vi "Instrument Manager Loop.vi"(8 "System Control":refnum<queue>, 11 "Instrument Manager":refnum<queue>) -> (0 "error out":errorcluster)   [LabVIEW 2020, in "plugin_flodx_pressure.lvlib" / "plugin.lvlib" / "Instrument Manager.lvlib"]
uses:
  Instrument Manager.lvlib
  <userlib>/RxnRover/PluginCore/src/support/Message Queue/Message Cluster.ctl
  Instrument Loop State.ctl
  connection_info/Connection Info.ctl
  Instrument State.ctl
  Instrument Config.ctl
  <vilib>/Utility/error.llb/Error Cluster From Error Code.vi
  <vilib>/ErrorRing/Error Ring.xnode
  <userlib>/RxnRover/PluginCore/src/support/Message Queue/Message Queue.lvlib
  <userlib>/_OpenG.lib/lvdata/lvdata.llb/openg_variant.lvlib
  mock_driver/mock_driver.lvlib
  <instrlib>/RxnRover/FloDx Pressure Driver/driver_flodx_pressure.lvlib
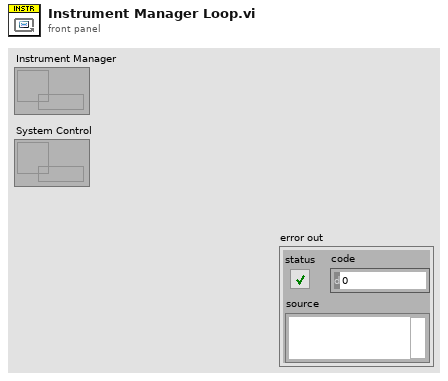
[diagram p1: front panel]
types:
  T1 = typedef "plugin_flodx_pressure.lvlib/plugin.lvlib/Instrument Manager.lvlib/Instrument Loop State.ctl" = cluster{"Connection Info":T2, "Running":bool, "Running Since":timestamp, "Instrument State":T3}
  T2 = typedef "plugin_flodx_pressure.lvlib/plugin.lvlib/Instrument Manager.lvlib/Connection Info.ctl" = cluster{"VISA Resource":refnum<visa-resource-name>, "Address":u8}
  T3 = typedef "plugin_flodx_pressure.lvlib/plugin.lvlib/Instrument Manager.lvlib/Instrument State.ctl" = cluster{"Abs. Pressure":sgl, "Amb. Pressure":sgl, "Device":string, "Firmware Version":string, "Error Status":bool, "Error Code":i32, "Error Source":string, "Gauge Pressure":sgl, "Temperature":sgl, "Units (0-kPa,1-PSI,2-BAR)":dbl}
  T4 = typedef "plugin_flodx_pressure.lvlib/plugin.lvlib/Instrument Manager.lvlib/Instrument Config.ctl" = cluster{"Device":string, "Firmware Version":string}
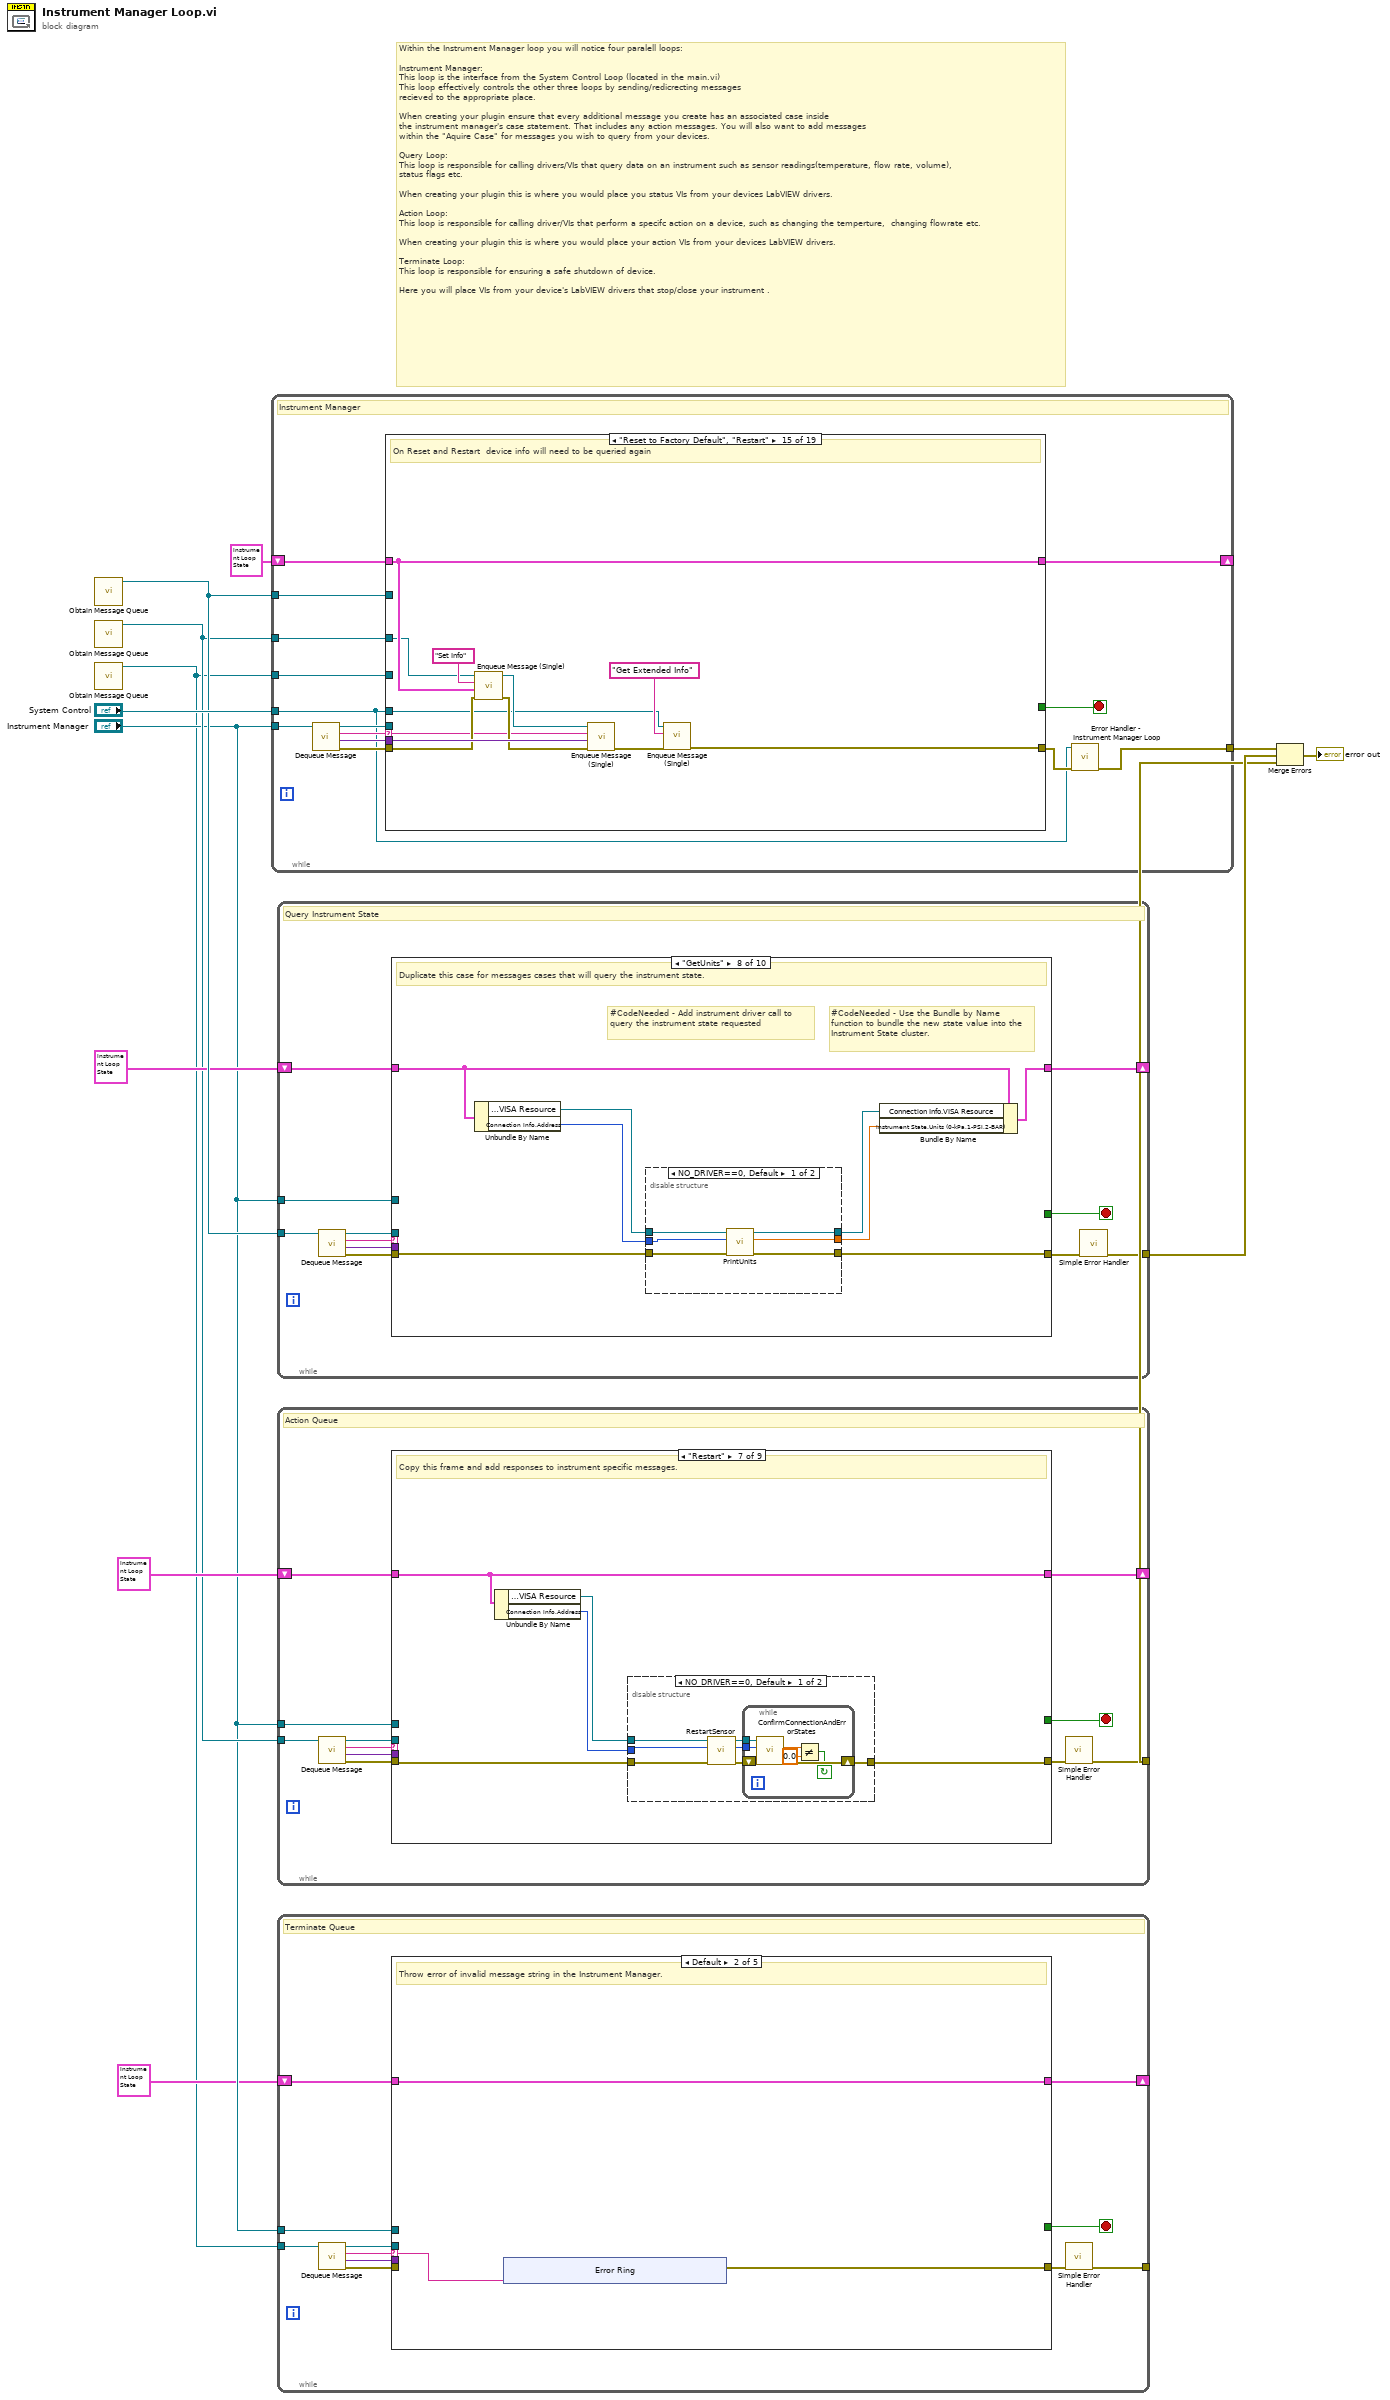
[diagram p0: block diagram]
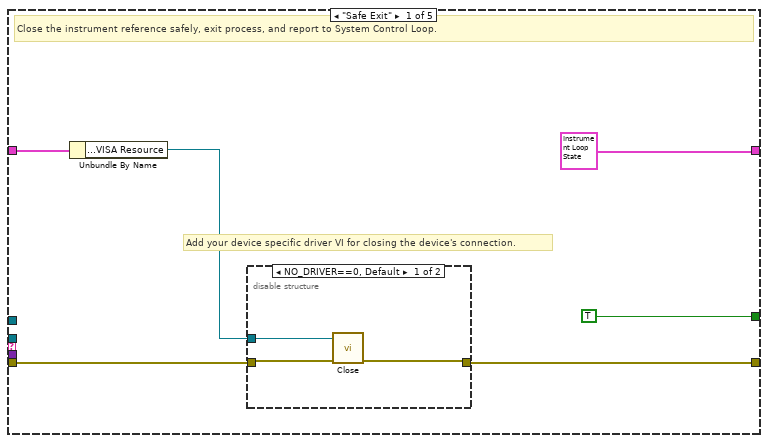
[diagram p2: hidden frame]
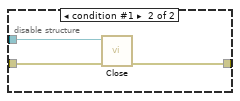
[diagram p3: hidden frame]
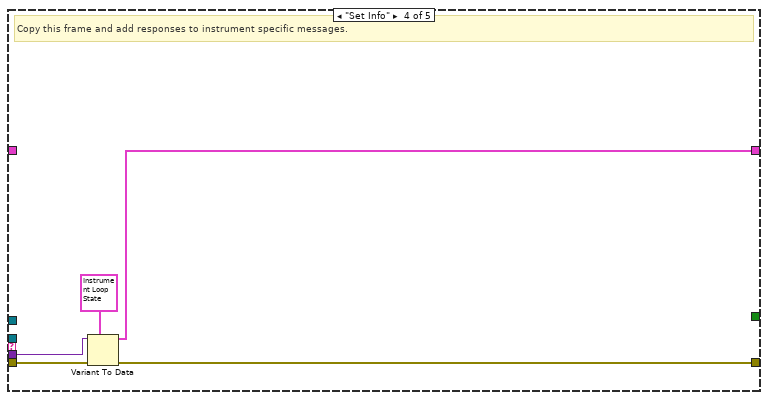
[diagram p5: hidden frame]
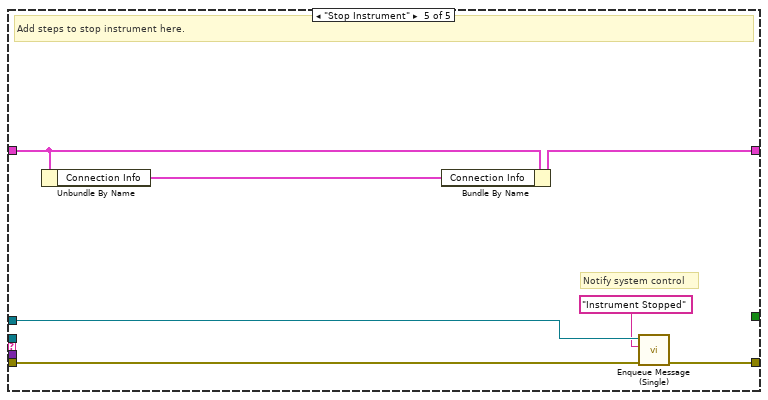
[diagram p6: hidden frame]
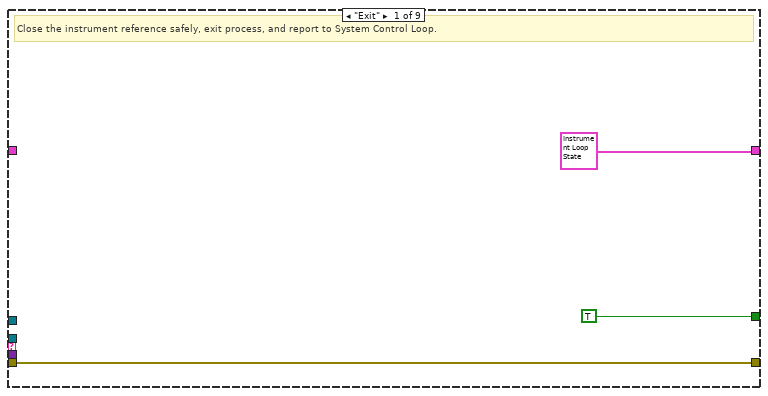
[diagram p7: hidden frame]
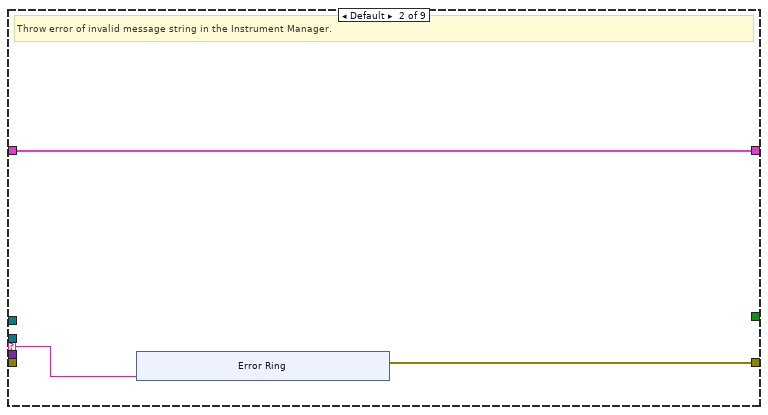
[diagram p8: hidden frame]
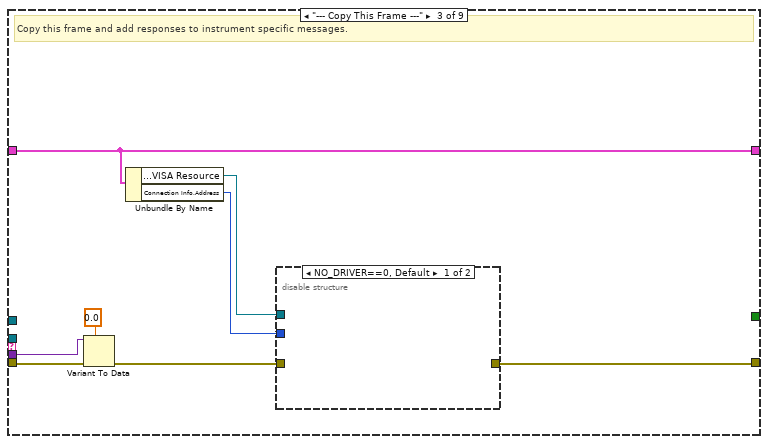
[diagram p9: hidden frame]
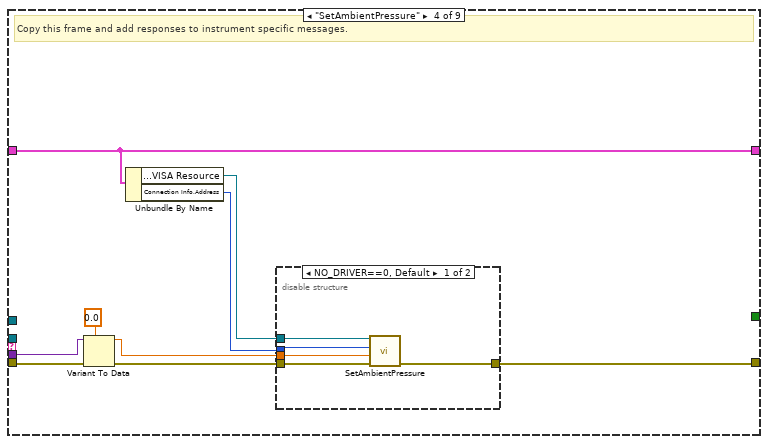
[diagram p11: hidden frame]
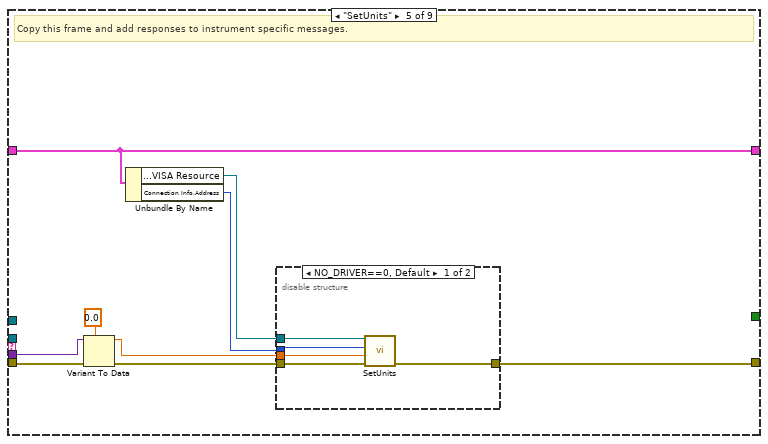
[diagram p13: hidden frame]
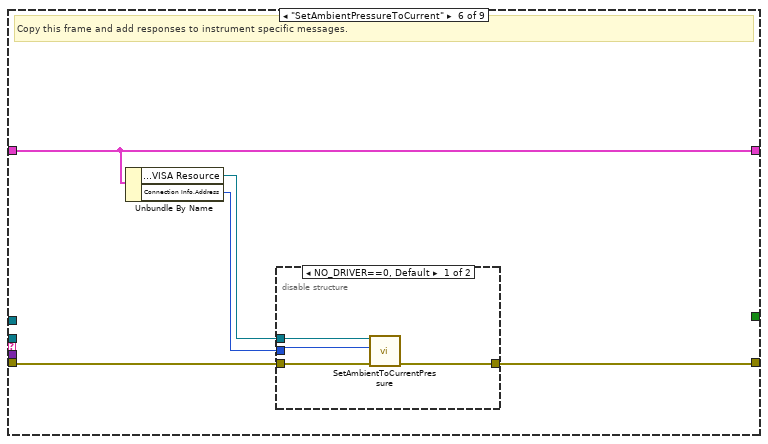
[diagram p15: hidden frame]
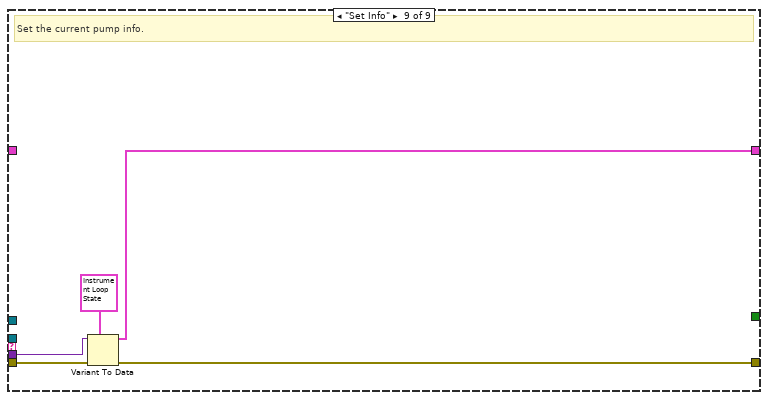
[diagram p19: hidden frame]
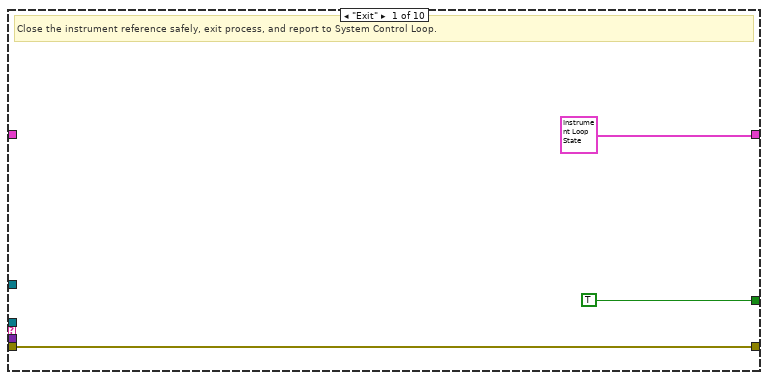
[diagram p20: hidden frame]
diagram:
  # "Within the Instrument Manager loop you will notice four paralell loops:\n\nInstrument Manager:\nThis loop is the interface from the System Control Loop (located in the main.vi)\nThis loop effectively controls the other three loops by sending/redicrecting messages\nrecieved to the appropriate place. \n\nWhen creating your plugin ensure that every additional message you create has an associated case inside \nthe instrument manager's case statement. That includes any action messages. You will also want to add messages\nwithin the \"Aquire Case\" for messages you wish to query from your devices.\n\nQuery Loop:\nThis loop is responsible for calling drivers/VIs that query data on an instrument such as sensor readings(temperature, flow rate, volume),\nstatus flags etc.\n\nWhen creating your plugin this is where you would place you status VIs from your devices LabVIEW drivers.\n\nAction Loop: \nThis loop is responsible for calling driver/VIs that perform a specifc action on a device, such as changing the temperture,  changing flowrate etc.\n\nWhen creating your plugin this is where you would place your action VIs from your devices LabVIEW drivers.\n\nTerminate Loop:\nThis loop is responsible for ensuring a safe shutdown of device. \n\nHere you will place VIs from your device's LabVIEW drivers that stop/close your instrument ."
  n1 = call <userlib>:"Obtain Message Queue.vi"() -> ("Message Queue"=w10:refnum<queue>)  [unwired: 10 in, 1 out]
  n2 = call <userlib>:"Obtain Message Queue.vi"() -> ("Message Queue"=w5:refnum<queue>)  [unwired: 10 in, 1 out]
  n3 = call <userlib>:"Obtain Message Queue.vi"() -> ("Message Queue"=w1:refnum<queue>)  [unwired: 10 in, 1 out]
  n4 = while {
    tunnel: "Instrument Manager" -> [w27]
    tunnel: "System Control" -> [w18]
    tunnel: [w21] -> w13
    shift-right: [w14] -> _
    shift-left: T1 {"Connection Info"={"VISA Resource"="", "Address"=1}, "Running"=FALSE, "Running Since"=timestamp(0 s since 1904-01-01), "Instrument State"={"Abs. Pressure"=0.0, "Amb. Pressure"=0.0, "Device"="", "Firmware Version"="", "Error Status"=FALSE, "Error Code"=0, "Error Source"="", "Gauge Pressure"=0.0, "Temperature"=0.0, "Units (0-kPa,1-PSI,2-BAR)"=0.0}} ("Default Instrument State") -> [w20]
    tunnel: w10 -> [w17]
    tunnel: w5 -> [w16]
    tunnel: w1 -> [w15]
    stop <- w19 stop-if-true
    # "Instrument Manager"
    n5 = call <userlib>:"Dequeue Message.vi"("Message Queue"=w27) -> ("error out"=w23:errorcluster, "Message Data"=w24:variant, "Message"=w26:string, "dup Message Queue"=w25:refnum<queue>)  [unwired: 7 in]
    n6 = case shown="\"Reset to Factory Default\", \"Restart\"" w26 {
      selector: w26 -> [_ w37 _ _ _ _ _ w83 _ _ w128 w132 w145 w154 w167 _ _ _ _]
      tunnel: w25 -> [w30 _ _ w54 _ _ _ _ _ w94 _ _ _ _ _ _ _ _ w206]
      tunnel: w18 -> [_ w38 _ _ w64 w74 w80 _ _ w96 w124 _ _ _ w162 _ _ _ _]
      tunnel: w24 -> [_ _ _ w61 _ _ _ _ _ w102 w127 w139 w151 w160 w173 _ _ _ w207]
      tunnel: w23 -> [w31 w39 w46 w59 w66 w71 w77 _ w92 w101 w126 w136 w148 w157 w170 w175 w176 w192 w212]
      tunnel: [w29 w33 w47 w56 w65 w75 w81 w82 w92 w105 w129 w140 w152 w161 w164 w175 w182 w202 w203] -> w22
      tunnel: w20 -> [_ w36 _ w60 w67 w69 w78 w84 w93 w104 w125 w137 w149 w158 w171 w174 w181 w199 w211]
      tunnel: [w32 w36 T1 {"Connection Info"={"VISA Resource"="", "Address"=1}, "Running"=FALSE, "Running Since"=timestamp(0 s since 1904-01-01), "Instrument State"={"Abs. Pressure"=0.0, "Amb. Pressure"=0.0, "Device"="", "Firmware Version"="", "Error Status"=FALSE, "Error Code"=0, "Error Source"="", "Gauge Pressure"=0.0, "Temperature"=0.0, "Units (0-kPa,1-PSI,2-BAR)"=0.0}} w60 w67 w69 w78 w84 w93 w103 w125 w131 w144 w158 w171 w174 w181 w199 w205] -> w14
      tunnel: [_ _ TRUE _ _ _ _ _ _ _ _ _ _ _ _ _ _ _ _] -> w19
      tunnel: w17 -> [_ _ w41 _ _ _ _ _ _ _ _ _ _ _ _ _ w180 w194 _]
      tunnel: w16 -> [_ _ w42 _ _ _ _ _ _ _ _ _ w141 w153 w166 _ _ _ _]
      tunnel: w15 -> [_ _ w43 _ _ _ _ _ _ _ _ w134 _ _ _ _ _ _ _]
      frame "Initialize" {
        (unwired) string[] ["Send Instrument Config", "Send Entry Names"]
        w32 = T1 {"Connection Info"={"VISA Resource"="", "Address"=1}, "Running"=FALSE, "Running Since"=timestamp(0 s since 1904-01-01), "Instrument State"={"Abs. Pressure"=0.0, "Amb. Pressure"=0.0, "Device"="", "Firmware Version"="", "Error Status"=FALSE, "Error Code"=0, "Error Source"="", "Gauge Pressure"=0.0, "Temperature"=0.0, "Units (0-kPa,1-PSI,2-BAR)"=0.0}}  # Default Instrument State
        # "Initialize the loop data."
        n7 = call <userlib>:"Enqueue Message (Array).vi"("error in (no error)"=w31, "Message Array"=string[] ["Send Instrument Config", "Send Acquisition Messages", "Send Entry Names"], "Message Queue"=w30) -> ("error out"=w29:errorcluster)  [unwired: 7 in, 1 out]
      }
      frame "Report" {
        # "Reports the instrument state to the system control loop to populate the rest of the plugin"
        # "Unblock querying"
        # "Report the instrument state."
        n8 = call <userlib>:"Enqueue Message (Single).vi"("error in (no error)"=w39, "Message Data"=w36, "Message"=w37, "Message Queue"=w38) -> ("error out"=w34:errorcluster)  [unwired: 6 in, 1 out]
        n9 = call "QueryInProgress.vi"("error in (no error)"=w34, "Action"=enum16{"Get", "Set False", "Set True"}."Set False") -> ("error out"=w33:errorcluster)  [unwired: 8 in, 1 out]
      }
      frame "Exit" {
        # "Close the instrument reference safely, exit process, and report to System Control Loop."
        n10 = Build Array(w41, w42) -> (w40:refnum<queue>[])
        n11 = call <userlib>:"Enqueue Message (Single).vi"("error in (no error)"=w46, "Message"="Safe Exit", "Message Queue"=w43) -> ("error out"=w45:errorcluster)  [unwired: 7 in, 1 out]
        n12 = for {
          tunnel: w40 -> [w52] mode=indexing
          tunnel: w45 -> [w50]
          tunnel: [w53] -> w47
          n13 = call <userlib>:"Enqueue Message (Single).vi"("error in (no error)"=w50, "Message"="Exit", "Message Queue"=w52) -> ("error out"=w53:errorcluster)  [unwired: 7 in, 1 out]
        }
      }
      frame "New Instrument Config" {
        # "No settings right now"
        # "If the new config is accepted, notify everything of the new values"
        # "Update the configs based on the user settings."
        n14 = Variant To Data(error in=w59, type=T4 {"Device"="", "Firmware Version"=""} ("Instrument Configuration"), Variant=w61) -> (error out=w55:errorcluster)  [unwired: 1 out]
        n15 = call <userlib>:"Enqueue Message (Single).vi"("error in (no error)"=w55, "Message"="Send Instrument Config", "Message Queue"=w54) -> ("error out"=w56:errorcluster)  [unwired: 7 in, 1 out]
      }
      frame "Send Instrument Config" {
        # "Send out the current values for the public loop configs."
        n16 = call <userlib>:"Enqueue Message (Single).vi"("error in (no error)"=w66, "Message Data"=T4 {"Device"="", "Firmware Version"=""} ("Instrument Configuration"), "Message"="Instrument Config", "Message Queue"=w64) -> ("error out"=w65:errorcluster)  [unwired: 6 in, 1 out]
      }
      frame "Send Entry Names" {
        # "#note: This is auto-populated based on the Instrument State TypeDef entry labels."
        # "Send the display names of entry values that will be reported by this instrument in each \"Report\" call."
        n17 = Unbundle By Name(w69) -> ("Instrument State"=w68:T3)
        n18 = call <userlib>:"Get Cluster Element Names__ogtk.vi"("error in (no error)"=w71, "Cluster"=w68) -> ("error out"=w70:errorcluster, "Element Names"=w72:string[])  [unwired: 8 in]
        n19 = call <userlib>:"Enqueue Message (Single).vi"("error in (no error)"=w70, "Message Data"=w72, "Message"="Set Entry Names", "Message Queue"=w74) -> ("error out"=w75:errorcluster)  [unwired: 6 in, 1 out]
      }
      frame "Send Acquisition Messages" {
        # "Send the messages that should be used to acquire the relevant instrument state and how to report it."
        n20 = call <userlib>:"Enqueue Message (Single).vi"("error in (no error)"=w77, "Message Data"=string[] ["Acquire"], "Message"="Set Acquisition Messages", "Message Queue"=w80) -> ("error out"=w81:errorcluster)  [unwired: 6 in, 1 out]
      }
      frame Default {
        # "Throw error of invalid message string in the Instrument Manager."
        n21 = xnode "Error Ring"("parameter 0"=w83) -> ("error out"=w82:errorcluster)
      }
      frame "--- Copy This Frame ---" {
        # "Copy this frame and add responses to instrument specific messages."
      }
      frame "Set Connection Info" {
        # "Validate and initialize the connection info"
        n22 = Variant To Data(error in=w101, type=T2 {"VISA Resource"="", "Address"=1} ("Connection Info"), Variant=w102) -> (data=w99:T2, error out=w100:errorcluster)
        n23 = call "Attempt Connection.vi"("error in (no error)"=w100, "Connection Info"=w99) -> ("error out"=w97:errorcluster, "Connection Info (duplicate)"=w98:T2)  [unwired: 8 in]
        n24 = case shown="No Error" w97 {
          selector: w97 -> [w107 w119]
          tunnel: w98 -> [w106 _]
          tunnel: [w108 w122] -> w105
          tunnel: w104 -> [w115 w123]
          tunnel: [w117 w123] -> w103
          tunnel: w96 -> [w116 w121]
          tunnel: w94 -> [w112 _]
          frame No Error {
            # "Notify System Control of valid connection info"
            # "Initialize valid resource."
            n25 = call <userlib>:"Enqueue Message (Single).vi"("error in (no error)"=w107, "Message Data"=w106, "Message"="Valid Connection Info", "Message Queue"=w116) -> ("error out"=w114:errorcluster)  [unwired: 6 in, 1 out]
            n26 = Bundle By Name(cluster=w115, "Connection Info"=w106) -> (w117:T1)
            n27 = call <userlib>:"Enqueue Message (Single).vi"("error in (no error)"=w114, "Message"="Send Acquisition Messages", "Message Queue"=w112) -> ("error out"=w109:errorcluster, "dup Message Queue"=w111:refnum<queue>)  [unwired: 7 in]
            n28 = call <userlib>:"Enqueue Message (Single).vi"("error in (no error)"=w109, "Message"="Get Extended Info", "Message Queue"=w111) -> ("error out"=w108:errorcluster)  [unwired: 7 in, 1 out]
          }
          frame Error {
            # "Report invalid resource."
            n29 = call <userlib>:"Enqueue Message (Single).vi"("Message Data"=w119, "Message"="Invalid Connection Info", "Message Queue"=w121) -> ("error out"=w122:errorcluster)  [unwired: 7 in, 1 out]
          }
        }
      }
      frame "Instrument Started", "Instrument Stopped" {
        # "Forward start/stop messages to the rest of the program."
        n30 = call <userlib>:"Enqueue Message (Single).vi"("error in (no error)"=w126, "Message Data"=w127, "Message"=w128, "Message Queue"=w124) -> ("error out"=w129:errorcluster)  [unwired: 6 in, 1 out]
      }
      frame "Stop Instrument" {
        # "Stop the instrument action."
        n31 = call <userlib>:"Enqueue Message (Single).vi"("error in (no error)"=w136, "Message Data"=w137, "Message"="Set Info", "Message Queue"=w134) -> ("error out"=w135:errorcluster, "dup Message Queue"=w133:refnum<queue>)  [unwired: 6 in]
        n32 = call <userlib>:"Enqueue Message (Single).vi"("error in (no error)"=w135, "Message Data"=w139, "Message"=w132, "Message Queue"=w133) -> ("error out"=w140:errorcluster)  [unwired: 6 in, 1 out]
        n33 = Bundle By Name(cluster=w137, "Running"=FALSE) -> (w131:T1)
      }
      frame "Start Instrument" {
        # "Start the instrument action."
        n34 = call <userlib>:"Enqueue Message (Single).vi"("error in (no error)"=w148, "Message Data"=w149, "Message"="Set Info", "Message Queue"=w141) -> ("error out"=w147:errorcluster, "dup Message Queue"=w146:refnum<queue>)  [unwired: 6 in]
        n35 = call <userlib>:"Enqueue Message (Single).vi"("error in (no error)"=w147, "Message Data"=w151, "Message"=w145, "Message Queue"=w146) -> ("error out"=w152:errorcluster)  [unwired: 6 in, 1 out]
        n36 = Get Date/Time In Seconds() -> (seconds since 1Jan1904=w142:timestamp)
        n37 = Bundle By Name(cluster=w149, "Running"=TRUE, "Running Since"=w142) -> (w144:T1)
      }
      frame "SetAmbientPressure", "SetAmbientPressureToCurrent", "SetUnits" {
        # "Actions to be forwarded to the Action loop"
        n38 = call <userlib>:"Enqueue Message (Single).vi"("error in (no error)"=w157, "Message Data"=w158, "Message"="Set Info", "Message Queue"=w153) -> ("error out"=w156:errorcluster, "dup Message Queue"=w155:refnum<queue>)  [unwired: 6 in]
        n39 = call <userlib>:"Enqueue Message (Single).vi"("error in (no error)"=w156, "Message Data"=w160, "Message"=w154, "Message Queue"=w155) -> ("error out"=w161:errorcluster)  [unwired: 6 in, 1 out]
      }
      frame "Reset to Factory Default", "Restart" {
        # "On Reset and Restart  device info will need to be queried again"
        n40 = call <userlib>:"Enqueue Message (Single).vi"("error in (no error)"=w170, "Message Data"=w171, "Message"="Set Info", "Message Queue"=w166) -> ("error out"=w169:errorcluster, "dup Message Queue"=w168:refnum<queue>)  [unwired: 6 in]
        n41 = call <userlib>:"Enqueue Message (Single).vi"("error in (no error)"=w169, "Message Data"=w173, "Message"=w167, "Message Queue"=w168) -> ("error out"=w165:errorcluster)  [unwired: 6 in, 1 out]
        n42 = call <userlib>:"Enqueue Message (Single).vi"("error in (no error)"=w165, "Message"="Get Extended Info", "Message Queue"=w162) -> ("error out"=w164:errorcluster)  [unwired: 7 in, 1 out]
      }
      frame "--- Copy for Get State Messages ---" {
        # "#CodeNeeded - Use the Bundle by Name function to bundle the new state value into the Instrument State cluster."
        # "#CodeNeeded - Add instrument driver call to query the instrument state requested"
        # "Duplicate this case for messages cases that will query the instrument state."
      }
      frame "Acquire" {
        # "Only query if there isn't another query in progress"
        # "Query the run state of the instrument."
        n43 = call "QueryInProgress.vi"("error in (no error)"=w176, "Action"=enum16{"Get", "Set False", "Set True"}."Get") -> ("error out"=w177:errorcluster, "Value"=w178:bool)  [unwired: 8 in]
        n44 = case shown="False" w178 {
          tunnel: w177 -> [w183 w191]
          tunnel: [w183 w190] -> w182
          tunnel: w181 -> [_ w187]
          tunnel: w180 -> [_ w185]
          frame True {
            # "There is another process inside Query Instrument\nstate, wait until it is finished"
          }
          frame False {
            # "replace this and add more\nif needed"
            n45 = call <userlib>:"Enqueue Message (Single).vi"("error in (no error)"=w191, "Message Data"=w187, "Message"="Set Info", "Message Queue"=w185) -> ("error out"=w188:errorcluster, "dup Message Queue"=w184:refnum<queue>)  [unwired: 6 in]
            n46 = call <userlib>:"Enqueue Message (Array).vi"("error in (no error)"=w188, "Message Array"=string[] ["GetGaugePressure", "GetAbsolutePressure", "GetTemperature", "Send Instr State"], "Message Queue"=w184) -> ("error out"=w190:errorcluster)  [unwired: 7 in, 1 out]
          }
        }
      }
      frame "Get Extended Info" {
        # "Add query messages to get\nimportant information but \nnot necessarilly required \nqueried constantly, such as\ndevice firmware information,\nname, etc."
        # "Block Aquire from querying"
        # "This is high priority, and is non-blocked from querying instrument state"
        # "This is information that is important but not necessarily required to be queried every time aquire message is sent"
        n47 = Flush Queue(queue=w194) -> (queue out=w193:refnum<queue>)  [unwired: 1 in, 2 out]
        n48 = call "QueryInProgress.vi"("error in (no error)"=w192, "Action"=enum16{"Get", "Set False", "Set True"}."Set True") -> ("error out"=w195:errorcluster)  [unwired: 8 in, 1 out]
        n49 = call <userlib>:"Enqueue Message (Single).vi"("error in (no error)"=w195, "Message Data"=w199, "Message"="Set Info", "Message Queue"=w193) -> ("error out"=w200:errorcluster, "dup Message Queue"=w197:refnum<queue>)  [unwired: 6 in]
        n50 = call <userlib>:"Enqueue Message (Array).vi"("error in (no error)"=w200, "Message Array"=string[] ["GetUnits", "GetAmbientPressure", "Send Instr State"], "Message Queue"=w197) -> ("error out"=w202:errorcluster)  [unwired: 7 in, 1 out]
      }
      frame "Set Instr State" {
        # "Set the new instrument state queried from the instrument."
        n51 = Variant To Data(error in=w212, type=T3 {"Abs. Pressure"=0.0, "Amb. Pressure"=0.0, "Device"="", "Firmware Version"="", "Error Status"=FALSE, "Error Code"=0, "Error Source"="", "Gauge Pressure"=0.0, "Temperature"=0.0, "Units (0-kPa,1-PSI,2-BAR)"=0.0} ("Instrument State"), Variant=w207) -> (data=w204:T3, error out=w209:errorcluster)
        n52 = Bundle By Name(cluster=w211, "Instrument State"=w204) -> (w205:T1)
        n53 = call <userlib>:"Enqueue Message (Single).vi"("error in (no error)"=w209, "Message"="Report", "Message Queue"=w206) -> ("error out"=w203:errorcluster)  [unwired: 7 in, 1 out]
      }
    }
    n54 = call "Error Handler - Instrument Manager Loop.vi"("error in (no error)"=w22, "Message Queue"=w18) -> ("dup error in"=w21:errorcluster)  [unwired: 8 in, 1 out]
  }
  n55 = while {
    tunnel: w10 -> [w223]
    shift-right: [w217] -> _
    shift-left: T1 {"Connection Info"={"VISA Resource"="", "Address"=1}, "Running"=FALSE, "Running Since"=timestamp(0 s since 1904-01-01), "Instrument State"={"Abs. Pressure"=0.0, "Amb. Pressure"=0.0, "Device"="", "Firmware Version"="", "Error Status"=FALSE, "Error Code"=0, "Error Source"="", "Gauge Pressure"=0.0, "Temperature"=0.0, "Units (0-kPa,1-PSI,2-BAR)"=0.0}} ("Default Instrument State") -> [w218]
    tunnel: "Instrument Manager" -> [w215]
    tunnel: [w213] -> w7
    stop <- w216 stop-if-true
    # "Query Instrument State"
    n56 = call <userlib>:"Dequeue Message.vi"("Message Queue"=w223) -> ("error out"=w219:errorcluster, "Message Data"=w220:variant, "Message"=w222:string, "dup Message Queue"=w221:refnum<queue>)  [unwired: 7 in]
    n57 = case shown="\"GetUnits\"" w222 {
      selector: w222 -> [_ w228 _ _ _ _ _ _ _ _]
      tunnel: w221 -> [_ _ _ _ _ _ _ _ _ _]
      tunnel: w220 -> [_ _ _ _ _ _ _ _ w331 _]
      tunnel: w219 -> [w224 _ w241 w250 w267 w284 w301 w318 w333 w339]
      tunnel: [w224 w227 w242 w251 w268 w285 w302 w319 w332 w334] -> w214
      tunnel: w218 -> [_ w229 w239 w248 w265 w282 w299 w316 _ w337]
      tunnel: [T1 {"Connection Info"={"VISA Resource"="", "Address"=1}, "Running"=FALSE, "Running Since"=timestamp(0 s since 1904-01-01), "Instrument State"={"Abs. Pressure"=0.0, "Amb. Pressure"=0.0, "Device"="", "Firmware Version"="", "Error Status"=FALSE, "Error Code"=0, "Error Source"="", "Gauge Pressure"=0.0, "Temperature"=0.0, "Units (0-kPa,1-PSI,2-BAR)"=0.0}} w229 w240 w249 w266 w283 w300 w317 w329 w337] -> w217
      tunnel: [TRUE _ _ _ _ _ _ _ _ _] -> w216
      tunnel: w215 -> [_ _ _ _ _ _ _ _ _ w338]
      frame "Exit" {
        # "Close the instrument reference safely, exit process, and report to System Control Loop."
      }
      frame Default {
        # "Throw error of invalid message string in the Instrument Manager."
        n58 = xnode "Error Ring"("parameter 0"=w228) -> ("error out"=w227:errorcluster)
      }
      frame "--- Copy for Get State Messages ---" {
        # "#CodeNeeded - Use the Bundle by Name function to bundle the new state value into the Instrument State cluster."
        # "#CodeNeeded - Add instrument driver call to query the instrument state requested"
        # "Duplicate this case for messages cases that will query the instrument state."
        n59 = Unbundle By Name(w239) -> ("Connection Info.VISA Resource"=w238:refnum<visa-resource-name>)  [unwired: 2 out]
        n60 = disable-structure shown="NO_DRIVER==0, Default" {
          disable-tunnel: w241 -> [_ w243]
          disable-tunnel: [_ w243] -> w242
          disable-tunnel: w238 -> [_ _]
          frame condition #0 (active) {
          }
          frame condition #1 {
          }
        }
        n61 = Bundle By Name(cluster=w239, "Instrument State"=T3 {"Abs. Pressure"=0.0, "Amb. Pressure"=0.0, "Device"="", "Firmware Version"="", "Error Status"=FALSE, "Error Code"=0, "Error Source"="", "Gauge Pressure"=0.0, "Temperature"=0.0, "Units (0-kPa,1-PSI,2-BAR)"=0.0}) -> (w240:T1)
      }
      frame "GetAmbientPressure" {
        # "#CodeNeeded - Use the Bundle by Name function to bundle the new state value into the Instrument State cluster."
        # "#CodeNeeded - Add instrument driver call to query the instrument state requested"
        # "Duplicate this case for messages cases that will query the instrument state."
        n62 = Unbundle By Name(w248) -> ("Connection Info.VISA Resource"=w247:refnum<visa-resource-name>, "Connection Info.Address"=w246:u8)
        n63 = disable-structure shown="NO_DRIVER==0, Default" {
          disable-tunnel: w250 -> [w256 w260]
          disable-tunnel: [w257 w260] -> w251
          disable-tunnel: w247 -> [w255 w259]
          disable-tunnel: w246 -> [w254 _]
          disable-tunnel: [w253 21.0 ("Ambient Pressure")] -> w245
          disable-tunnel: [w252 w259] -> w244
          frame condition #0 (active) {
            n64 = call <instrlib>:"PrintAmbientPressure.vi"("error in (no error)"=w256, "Address"=w254, "VISA resource name"=w255) -> ("error out"=w257:errorcluster, "Ambient Pressure"=w253:dbl, "VISA resource name out"=w252:refnum<visa-resource-name>)  [unwired: 5 in, 1 out]
          }
          frame condition #1 {
          }
        }
        n65 = Bundle By Name(cluster=w248, "Connection Info.VISA Resource"=w244, "Instrument State.Amb. Pressure"=w245) -> (w249:T1)
      }
      frame "GetAbsolutePressure" {
        # "#CodeNeeded - Use the Bundle by Name function to bundle the new state value into the Instrument State cluster."
        # "#CodeNeeded - Add instrument driver call to query the instrument state requested"
        # "Duplicate this case for messages cases that will query the instrument state."
        n66 = Unbundle By Name(w265) -> ("Connection Info.VISA Resource"=w264:refnum<visa-resource-name>, "Connection Info.Address"=w263:u8)
        n67 = disable-structure shown="NO_DRIVER==0, Default" {
          disable-tunnel: w267 -> [w273 w277]
          disable-tunnel: [w274 w277] -> w268
          disable-tunnel: w264 -> [w272 w276]
          disable-tunnel: w263 -> [w271 _]
          disable-tunnel: [w270 21.0 ("Ambient Pressure")] -> w262
          disable-tunnel: [w269 w276] -> w261
          frame condition #0 (active) {
            n68 = call <instrlib>:"PrintAbsolutePressure.vi"("error in (no error)"=w273, "Address"=w271, "VISA resource name"=w272) -> ("error out"=w274:errorcluster, "Abs. Pressure"=w270:dbl, "VISA resource name out"=w269:refnum<visa-resource-name>)  [unwired: 5 in, 1 out]
          }
          frame condition #1 {
          }
        }
        n69 = Bundle By Name(cluster=w265, "Connection Info.VISA Resource"=w261, "Instrument State.Abs. Pressure"=w262) -> (w266:T1)
      }
      frame "GetGaugePressure" {
        # "#CodeNeeded - Use the Bundle by Name function to bundle the new state value into the Instrument State cluster."
        # "#CodeNeeded - Add instrument driver call to query the instrument state requested"
        # "Duplicate this case for messages cases that will query the instrument state."
        n70 = Unbundle By Name(w282) -> ("Connection Info.VISA Resource"=w281:refnum<visa-resource-name>, "Connection Info.Address"=w280:u8)
        n71 = disable-structure shown="NO_DRIVER==0, Default" {
          disable-tunnel: w284 -> [w290 w294]
          disable-tunnel: [w291 w294] -> w285
          disable-tunnel: w281 -> [w289 w293]
          disable-tunnel: w280 -> [w288 _]
          disable-tunnel: [w287 21.0 ("Ambient Pressure")] -> w279
          disable-tunnel: [w286 w293] -> w278
          frame condition #0 (active) {
            n72 = call <instrlib>:"PrintGaugePresssure.vi"("error in (no error)"=w290, "Address"=w288, "VISA resource name"=w289) -> ("error out"=w291:errorcluster, "Print Gauge Pressure"=w287:dbl, "VISA resource name out"=w286:refnum<visa-resource-name>)  [unwired: 5 in, 1 out]
          }
          frame condition #1 {
          }
        }
        n73 = Bundle By Name(cluster=w282, "Connection Info.VISA Resource"=w278, "Instrument State.Gauge Pressure"=w279) -> (w283:T1)
      }
      frame "GetTemperature" {
        # "#CodeNeeded - Use the Bundle by Name function to bundle the new state value into the Instrument State cluster."
        # "#CodeNeeded - Add instrument driver call to query the instrument state requested"
        # "Duplicate this case for messages cases that will query the instrument state."
        n74 = Unbundle By Name(w299) -> ("Connection Info.VISA Resource"=w298:refnum<visa-resource-name>, "Connection Info.Address"=w297:u8)
        n75 = disable-structure shown="NO_DRIVER==0, Default" {
          disable-tunnel: w301 -> [w307 w311]
          disable-tunnel: [w308 w311] -> w302
          disable-tunnel: w298 -> [w306 w310]
          disable-tunnel: w297 -> [w305 _]
          disable-tunnel: [w304 21.0 ("Ambient Pressure")] -> w296
          disable-tunnel: [w303 w310] -> w295
          frame condition #0 (active) {
            n76 = call <instrlib>:"PrintTemperature.vi"("error in (no error)"=w307, "Address"=w305, "VISA resource name"=w306) -> ("error out"=w308:errorcluster, "Temperature"=w304:dbl, "VISA resource name out"=w303:refnum<visa-resource-name>)  [unwired: 5 in, 1 out]
          }
          frame condition #1 {
          }
        }
        n77 = Bundle By Name(cluster=w299, "Connection Info.VISA Resource"=w295, "Instrument State.Temperature"=w296) -> (w300:T1)
      }
      frame "GetUnits" {
        # "#CodeNeeded - Use the Bundle by Name function to bundle the new state value into the Instrument State cluster."
        # "#CodeNeeded - Add instrument driver call to query the instrument state requested"
        # "Duplicate this case for messages cases that will query the instrument state."
        n78 = Unbundle By Name(w316) -> ("Connection Info.VISA Resource"=w315:refnum<visa-resource-name>, "Connection Info.Address"=w314:u8)
        n79 = disable-structure shown="NO_DRIVER==0, Default" {
          disable-tunnel: w318 -> [w324 w328]
          disable-tunnel: [w325 w328] -> w319
          disable-tunnel: w315 -> [w323 w327]
          disable-tunnel: w314 -> [w322 _]
          disable-tunnel: [w321 21.0 ("Ambient Pressure")] -> w313
          disable-tunnel: [w320 w327] -> w312
          frame condition #0 (active) {
            n80 = call <instrlib>:"PrintUnits.vi"("error in (no error)"=w324, "Address"=w322, "VISA resource name"=w323) -> ("error out"=w325:errorcluster, "Units(0-Kpa,1-PSI,2-BAR)"=w321:dbl, "VISA resource name out"=w320:refnum<visa-resource-name>)  [unwired: 5 in, 1 out]
          }
          frame condition #1 {
          }
        }
        n81 = Bundle By Name(cluster=w316, "Connection Info.VISA Resource"=w312, "Instrument State.Units (0-kPa,1-PSI,2-BAR)"=w313) -> (w317:T1)
      }
      frame "Set Info" {
        # "Sets the instrument loop info needed for operation."
        n82 = Variant To Data(error in=w333, type=T1 {"Connection Info"={"VISA Resource"="", "Address"=1}, "Running"=FALSE, "Running Since"=timestamp(0 s since 1904-01-01), "Instrument State"={"Abs. Pressure"=0.0, "Amb. Pressure"=0.0, "Device"="", "Firmware Version"="", "Error Status"=FALSE, "Error Code"=0, "Error Source"="", "Gauge Pressure"=0.0, "Temperature"=0.0, "Units (0-kPa,1-PSI,2-BAR)"=0.0}} ("Default Instrument State"), Variant=w331) -> (data=w329:T1, error out=w332:errorcluster)
      }
      frame "Send Instr State" {
        # "Send the instrument state back to the control loop."
        n83 = Unbundle By Name(w337) -> ("Instrument State"=w336:T3)
        n84 = call <userlib>:"Enqueue Message (Single).vi"("error in (no error)"=w339, "Message Data"=w336, "Message"="Set Instr State", "Message Queue"=w338) -> ("error out"=w334:errorcluster)  [unwired: 6 in, 1 out]
      }
    }
    n85 = call <vilib>:"Simple Error Handler.vi"("error in (no error)"=w214) -> ("error out"=w213:errorcluster)  [unwired: 4 in, 4 out]
  }
  n86 = while {
    tunnel: w5 -> [w350]
    tunnel: "Instrument Manager" -> [w341]
    tunnel: [w340] -> w4
    shift-right: [w343] -> _
    shift-left: T1 {"Connection Info"={"VISA Resource"="", "Address"=1}, "Running"=FALSE, "Running Since"=timestamp(0 s since 1904-01-01), "Instrument State"={"Abs. Pressure"=0.0, "Amb. Pressure"=0.0, "Device"="", "Firmware Version"="", "Error Status"=FALSE, "Error Code"=0, "Error Source"="", "Gauge Pressure"=0.0, "Temperature"=0.0, "Units (0-kPa,1-PSI,2-BAR)"=0.0}} ("Default Instrument State") -> [w344]
    stop <- w342 stop-if-true
    # "Action Queue"
    n87 = call <userlib>:"Dequeue Message.vi"("Message Queue"=w350) -> ("error out"=w346:errorcluster, "Message Data"=w347:variant, "Message"=w349:string, "dup Message Queue"=w348:refnum<queue>)  [unwired: 7 in]
    n88 = case shown="\"Restart\"" w349 {
      selector: w349 -> [_ w355 _ _ _ _ _ _ _]
      tunnel: w348 -> [_ _ _ _ _ _ _ _ _]
      tunnel: w341 -> [_ _ _ _ _ _ _ _ _]
      tunnel: w347 -> [_ _ w368 w378 w393 _ _ _ w435]
      tunnel: w346 -> [w351 _ w369 w379 w394 w403 w413 w432 w437]
      tunnel: [w351 w354 w364 w374 w389 w404 w414 w432 w436] -> w345
      tunnel: w344 -> [_ w356 w371 w381 w396 w407 w417 w433 _]
      tunnel: [T1 {"Connection Info"={"VISA Resource"="", "Address"=1}, "Running"=FALSE, "Running Since"=timestamp(0 s since 1904-01-01), "Instrument State"={"Abs. Pressure"=0.0, "Amb. Pressure"=0.0, "Device"="", "Firmware Version"="", "Error Status"=FALSE, "Error Code"=0, "Error Source"="", "Gauge Pressure"=0.0, "Temperature"=0.0, "Units (0-kPa,1-PSI,2-BAR)"=0.0}} w356 w371 w381 w396 w407 w417 w433 w434] -> w343
      tunnel: [TRUE _ _ _ _ _ _ _ _] -> w342
      frame "Exit" {
        # "Close the instrument reference safely, exit process, and report to System Control Loop."
      }
      frame Default {
        # "Throw error of invalid message string in the Instrument Manager."
        n89 = xnode "Error Ring"("parameter 0"=w355) -> ("error out"=w354:errorcluster)
      }
      frame "--- Copy This Frame ---" {
        # "Copy this frame and add responses to instrument specific messages."
        n90 = Variant To Data(error in=w369, type=sgl 0.0, Variant=w368) -> (error out=w370:errorcluster)  [unwired: 1 out]
        n91 = Unbundle By Name(w371) -> ("Connection Info.VISA Resource"=w366:refnum<visa-resource-name>, "Connection Info.Address"=w365:u8)
        n92 = disable-structure shown="NO_DRIVER==0, Default" {
          disable-tunnel: w370 -> [_ w372]
          disable-tunnel: [_ w372] -> w364
          disable-tunnel: w366 -> [_ _]
          disable-tunnel: w365 -> [_ _]
          frame condition #0 (active) {
          }
          frame condition #1 {
          }
        }
      }
      frame "SetAmbientPressure" {
        # "Copy this frame and add responses to instrument specific messages."
        n93 = Variant To Data(error in=w379, type=sgl 0.0, Variant=w378) -> (data=w373:sgl, error out=w380:errorcluster)
        n94 = Unbundle By Name(w381) -> ("Connection Info.VISA Resource"=w376:refnum<visa-resource-name>, "Connection Info.Address"=w375:u8)
        n95 = disable-structure shown="NO_DRIVER==0, Default" {
          disable-tunnel: w380 -> [w385 w387]
          disable-tunnel: [w386 w387] -> w374
          disable-tunnel: w376 -> [w384 _]
          disable-tunnel: w375 -> [w383 _]
          disable-tunnel: w373 -> [w382 _]
          frame condition #0 (active) {
            n96 = call <instrlib>:"SetAmbientPressure.vi"("error in (no error)"=w385, "Ambient Pressure"=w382, "Address"=w383, "VISA resource name"=w384) -> ("error out"=w386:errorcluster)  [unwired: 5 in, 2 out]
          }
          frame condition #1 {
          }
        }
      }
      frame "SetUnits" {
        # "Copy this frame and add responses to instrument specific messages."
        n97 = Variant To Data(error in=w394, type=sgl 0.0, Variant=w393) -> (data=w388:sgl, error out=w395:errorcluster)
        n98 = Unbundle By Name(w396) -> ("Connection Info.VISA Resource"=w391:refnum<visa-resource-name>, "Connection Info.Address"=w390:u8)
        n99 = disable-structure shown="NO_DRIVER==0, Default" {
          disable-tunnel: w395 -> [w400 w402]
          disable-tunnel: [w401 w402] -> w389
          disable-tunnel: w391 -> [w399 _]
          disable-tunnel: w390 -> [w398 _]
          disable-tunnel: w388 -> [w397 _]
          frame condition #0 (active) {
            n100 = call <instrlib>:"SetUnits.vi"("error in (no error)"=w400, "Unit(0-kPa,1-PSI,2-BAR)"=w397, "Address"=w398, "VISA resource name"=w399) -> ("error out"=w401:errorcluster)  [unwired: 5 in, 2 out]
          }
          frame condition #1 {
          }
        }
      }
      frame "SetAmbientPressureToCurrent" {
        # "Copy this frame and add responses to instrument specific messages."
        n101 = Unbundle By Name(w407) -> ("Connection Info.VISA Resource"=w406:refnum<visa-resource-name>, "Connection Info.Address"=w405:u8)
        n102 = disable-structure shown="NO_DRIVER==0, Default" {
          disable-tunnel: w403 -> [w410 w412]
          disable-tunnel: [w411 w412] -> w404
          disable-tunnel: w406 -> [w409 _]
          disable-tunnel: w405 -> [w408 _]
          frame condition #0 (active) {
            n103 = call <instrlib>:"SetAmbientToCurrentPressure.vi"("error in (no error)"=w410, "Address"=w408, "VISA resource name"=w409) -> ("error out"=w411:errorcluster)  [unwired: 6 in, 2 out]
          }
          frame condition #1 {
          }
        }
      }
      frame "Restart" {
        # "Copy this frame and add responses to instrument specific messages."
        n104 = Unbundle By Name(w417) -> ("Connection Info.VISA Resource"=w416:refnum<visa-resource-name>, "Connection Info.Address"=w415:u8)
        n105 = disable-structure shown="NO_DRIVER==0, Default" {
          disable-tunnel: w413 -> [w423 w431]
          disable-tunnel: [w419 w431] -> w414
          disable-tunnel: w416 -> [w422 _]
          disable-tunnel: w415 -> [w418 _]
          frame condition #0 (active) {
            n106 = call <instrlib>:"RestartSensor.vi"("error in (no error)"=w423, "Address"=w418, "VISA resource name"=w422) -> ("error out"=w421:errorcluster, "VISA resource name out"=w420:refnum<visa-resource-name>)  [unwired: 7 in]
            n107 = while {
              tunnel: w420 -> [w429]
              shift-right: [w428] -> w419
              shift-left: w421 -> [w430]
              tunnel: w418 -> [w424]
              stop <- w427 continue-if-true
              n108 = call <instrlib>:"ConfirmConnectionAndErrorStates.vi"("error in (no error)"=w430, "Address"=w424, "VISA resource name"=w429) -> ("error out"=w428:errorcluster, "Value"=w426:dbl)  [unwired: 5 in, 2 out]
              n109 = Not Equal?(x=w426, y=0.0) -> (x != y?=w427:bool)
            }
          }
          frame condition #1 {
          }
        }
      }
      frame "Start Instrument" {
      }
      frame "Set Info" {
        # "Set the current pump info."
        n110 = Variant To Data(error in=w437, type=T1 {"Connection Info"={"VISA Resource"="", "Address"=1}, "Running"=FALSE, "Running Since"=timestamp(0 s since 1904-01-01), "Instrument State"={"Abs. Pressure"=0.0, "Amb. Pressure"=0.0, "Device"="", "Firmware Version"="", "Error Status"=FALSE, "Error Code"=0, "Error Source"="", "Gauge Pressure"=0.0, "Temperature"=0.0, "Units (0-kPa,1-PSI,2-BAR)"=0.0}} ("Default Instrument State"), Variant=w435) -> (data=w434:T1, error out=w436:errorcluster)
      }
    }
    n111 = call <vilib>:"Simple Error Handler.vi"("error in (no error)"=w345) -> ("error out"=w340:errorcluster)  [unwired: 4 in, 4 out]
  }
  n112 = while {
    tunnel: "Instrument Manager" -> [w441]
    tunnel: [w440] -> _
    shift-right: [w443] -> _
    shift-left: T1 {"Connection Info"={"VISA Resource"="", "Address"=1}, "Running"=FALSE, "Running Since"=timestamp(0 s since 1904-01-01), "Instrument State"={"Abs. Pressure"=0.0, "Amb. Pressure"=0.0, "Device"="", "Firmware Version"="", "Error Status"=FALSE, "Error Code"=0, "Error Source"="", "Gauge Pressure"=0.0, "Temperature"=0.0, "Units (0-kPa,1-PSI,2-BAR)"=0.0}} ("Default Instrument State") -> [w444]
    tunnel: w1 -> [w439]
    stop <- w442 stop-if-true
    # "Terminate Queue"
    n113 = call <userlib>:"Dequeue Message.vi"("Message Queue"=w439) -> ("error out"=w446:errorcluster, "Message Data"=w447:variant, "Message"=w449:string, "dup Message Queue"=w448:refnum<queue>)  [unwired: 7 in]
    n114 = case shown="Default" w449 {
      selector: w449 -> [_ w463 _ _ _]
      tunnel: w448 -> [_ _ _ _ _]
      tunnel: w441 -> [_ _ _ _ w484]
      tunnel: w447 -> [_ _ _ w475 _]
      tunnel: w446 -> [w452 _ w472 w477 w482]
      tunnel: [w451 w462 w472 w476 w485] -> w445
      tunnel: w444 -> [w455 w464 w473 _ w481]
      tunnel: [T1 {"Connection Info"={"VISA Resource"="", "Address"=1}, "Running"=FALSE, "Running Since"=timestamp(0 s since 1904-01-01), "Instrument State"={"Abs. Pressure"=0.0, "Amb. Pressure"=0.0, "Device"="", "Firmware Version"="", "Error Status"=FALSE, "Error Code"=0, "Error Source"="", "Gauge Pressure"=0.0, "Temperature"=0.0, "Units (0-kPa,1-PSI,2-BAR)"=0.0}} w464 w473 w474 w483] -> w443
      tunnel: [TRUE _ _ _ _] -> w442
      frame "Safe Exit" {
        # "Add your device specific driver VI for closing the device's connection."
        # "Close the instrument reference safely, exit process, and report to System Control Loop."
        n115 = Unbundle By Name(w455) -> ("Connection Info.VISA Resource"=w450:refnum<visa-resource-name>)
        n116 = disable-structure shown="NO_DRIVER==0, Default" {
          disable-tunnel: w452 -> [w457 w461]
          disable-tunnel: [w458 w460] -> w451
          disable-tunnel: w450 -> [w456 w459]
          frame condition #0 (active) {
            n117 = call <instrlib>:"Close.vi"("error in (no error)"=w457, "VISA resource name"=w456) -> ("error out"=w458:errorcluster)  [unwired: 9 in]
          }
          frame condition #1 {
            n118 = call <instrlib>:"Close.vi"("Error in"=w461, "VISA resource name"=w459) -> ("Error out"=w460:errorcluster)  [unwired: 9 in]
          }
        }
      }
      frame Default {
        # "Throw error of invalid message string in the Instrument Manager."
        n119 = xnode "Error Ring"("parameter 0"=w463) -> ("error out"=w462:errorcluster)
      }
      frame "--- Copy This Frame ---" {
        # "Copy this frame and add responses to instrument specific messages."
      }
      frame "Set Info" {
        # "Copy this frame and add responses to instrument specific messages."
        n120 = Variant To Data(error in=w477, type=T1 {"Connection Info"={"VISA Resource"="", "Address"=1}, "Running"=FALSE, "Running Since"=timestamp(0 s since 1904-01-01), "Instrument State"={"Abs. Pressure"=0.0, "Amb. Pressure"=0.0, "Device"="", "Firmware Version"="", "Error Status"=FALSE, "Error Code"=0, "Error Source"="", "Gauge Pressure"=0.0, "Temperature"=0.0, "Units (0-kPa,1-PSI,2-BAR)"=0.0}} ("Default Instrument State"), Variant=w475) -> (data=w474:T1, error out=w476:errorcluster)
      }
      frame "Stop Instrument" {
        # "Notify system control"
        # "Add steps to stop instrument here."
        n121 = Unbundle By Name(w481) -> ("Connection Info"=w480:T2)
        n122 = Bundle By Name(cluster=w481, "Connection Info"=w480) -> (w483:T1)
        n123 = call <userlib>:"Enqueue Message (Single).vi"("error in (no error)"=w482, "Message"="Instrument Stopped", "Message Queue"=w484) -> ("error out"=w485:errorcluster)  [unwired: 7 in, 1 out]
      }
    }
    n124 = call <vilib>:"Simple Error Handler.vi"("error in (no error)"=w445) -> ("error out"=w440:errorcluster)  [unwired: 4 in, 4 out]
  }
  n125 = Merge Errors(w13, w7, w4) -> (→"error out":errorcluster)
